vi "시리얼 테스트.vi"(11 "Serial Port":refnum<visa-resource-name>="COM6") -> ()   [LabVIEW 2015]
doc: "Use this template to create an application that executes repeatedly until you click the Stop button. This template polls the state of the Stop button and does not use events. Use the Top-Level Application template (not available in the Base package) to create a single-loop application with event handling."
uses:
  <vilib>/Utility/config.llb/Read Key (String).vi
  <vilib>/Utility/config.llb/Read Key (U32).vi
  <vilib>/Utility/config.llb/Read Key (Double).vi
  <vilib>/Utility/config.llb/Read Key (Boolean).vi
  <vilib>/Instr/_visa.llb/VISA Configure Serial Port (Instr).vi
  <vilib>/Utility/config.llb/Write Key (String).vi
  <vilib>/Utility/config.llb/Write Key (I32).vi
  <vilib>/Utility/config.llb/Write Key (Double).vi
  <vilib>/Utility/config.llb/Write Key (Boolean).vi
  <vilib>/Utility/config.llb/NI_LVConfig.lvlib
panel:
  out "수신 플래그":bool
  out "수신 버퍼 배열":u8[](array[numeric])=[79, 75, 43, 68, 73, 83, 67, 83, 79, 75, 43, 68, 73, 83, 51, 58, 54, 70, 55, 56, 55, 52, 54, 56, 50, 54, 57, 67, 79, 75, 43, 78, 65, 77, 69, 58, 71, 13, 10, 79, 75, 43, 68, 73, 83, 67, 69, 79, 75, 43, 68, 73, 83, 67, 83, 79, 75, 43, 68, 73, 83, 49, 58, 69, 50, 67, 70, 55, 57, 67, 69, 54, 68, 48, 49, 79, 75, 43, 78, 65, 77, 69, 58, 79, 117, 114, 67, 104, 97, 114, 97, 99, 116, 101, 114, 105, 115, 116, 105, 13, 10, 79, 75, 43, 68, 73, 83, 67, 69, 79, 75, 43, 68, 73, 83, 67, 83, 79, 75, 43, 68, 73, 83, 49, 58, 69, 50, 67, 70, 55, 57, 67, 69, 54, 68, 48, 49, 79, 75, 43, 78, 65, 77, 69, 58, 79, 117, 114, 67, 104, 97, 114, 97, 99, 116, 101, 114, 105, 115, 116, 105, 13, 10, 79, 75, 43, 68, 73, 83, 67, 69, 79, 75, 43, 71, 101, 116, 58, 48, 120, 70, 70, 69, 48, 79, 75, 43, 83, 101, 116, 58, 48, 120, 70, 48, 48, 68, 79, 75, 43, 71, 101, 116, 58, 48, 120, 70, 48, 48, 68, 79, 75, 43, 68, 73, 83, 73, 83, 79, 75, 43, 68, 73, 83, 67, 58, 48, 48, 48, 48, 48, 48, 48, 48, 58, 48, 48, 48, 48, 48, 48, 48, 48, 48, 48, 48, 48, 48, 48, 48, 48, 48, 48, 48, 48, 48, 48, 48, 48, 48, 48, 48, 48, 48, 48, 48, 48, 58, 48, 48, 48, 48, 48, 48, 48, 48, 48, 48, 58, 69, 50, 67, 70, 55, 57, 67, 69, 54, 68, 48, 49, 58, 45, 48, 51, 54, 79, 75, 43, 68, 73, 83, 67, 58, 48, 48, 48, 48, 48, 48, 48, 48, 58, 48, 48, 48, 48, 48, 48, 48, 48, 48, 48, 48, 48, 48, 48, 48, 48, 48, 48, 48, 48, 48, 48, 48, 48, 48, 48, 48, 48, 48, 48, 48, 48, 58, 48, 48, 48, 48, 48, 48, 48, 48, 48, 48, 58, 69, 50, 67, 70, 55, 57, 67, 69, 54, 68, 48, 49, 58, 45, 48, 51, 54, 79, 75, 43, 68, 73, 83, 67, 69, 79, 75, 43, 68, 73, 83, 67, 83, 79, 75, 43, 68, 73, 83, 49, 58, 69, 50, 67, 70, 55, 57, 67, 69, 54, 68, 48, 49, 79, 75, 43, 78, 65, 77, 69, 58, 79, 117, 114, 67, 104, 97, 114, 97, 99, 116, 101, 114, 105, 115, 116, 105, 13, 10, 79, 75, 43, 68, 73, 83, 67, 69, 79, 75, 43, 67, 79, 78, 78, 48, 79, 75, 43, 67, 79, 78, 78, 79, 75, 43, 76, 79, 83, 84, 79, 75, 79, 75, 79, 75]
  in  "Serial Port 동작":refnum<visa-resource-name>="COM6"
  in  "수신 텍스트 속성":enum16{"Normal", "'\\' code", "Password", "Hex"}(ring) caption="Display Style"
  in  "Pause":bool
  in  "Transmit New line":enum16{"None", "LF", "CR", "CR+LF"}(ring)
  in  "Baudrate(BPS)":T1(ring)=enum."9600"
  out "연속전송 타이머":u64=18183062
  in  "Interval(s)":dbl(slide)=0.1 min=0.001 max=5.0 step=0.001 scale=0.1..5.0
  in  "Clear":bool
  in  "포트 연결":bool=TRUE
  in  "TxD 14":string="aaaaaaa"
  in  "연속전송 1":bool
  in  "TxD 13":string="AT+CO1E2CF79CE6D01"
  in  "전송 13":bool
  in  "TxD 12":string="AT+CONN2"
  in  "전송 12":bool
  in  "TxD 11":string="AT+CONN0"
  in  "전송 11":bool
  in  "TxD 10":string="AT+DISI?"
  in  "전송 10":bool
  in  "TxD 9":string="AT+DISC?"
  in  "전송 9":bool
  in  "TxD 8":string="AT+VERS?"
  in  "전송 8":bool
  in  "TxD 7":string="AT+UUID?"
  in  "전송 7":bool
  in  "TxD 6":string="AT+UUID0xF00D"
  in  "전송 6":bool
  in  "TxD 5":string="AT+IBEA1"
  in  "전송 5":bool
  in  "TxD 4":string="AT+SHOW1"
  in  "전송 4":bool
  in  "TxD 3":string="AT+ROLE1"
  in  "전송 3":bool
  in  "TxD 2":string="AT+IMME1"
  in  "전송 2":bool
  in  "전송 1":bool
  in  "TxD 1":string="AT"
  in  "Program Exit":bool=TRUE
  out "Receive data":string="OK+DISCSOK+DIS3:6F787468269COK+NAME:G\r\nOK+DISCEOK+DISCSOK+DIS1:E2CF79CE6D01OK+NAME:OurCharacteristi\r\nOK+DISCEOK+DISCSOK+DIS1:E2CF79CE6D01OK+NAME:OurCharacteristi\r\nOK+DISCEOK+Get:0xFFE0OK+Set:0xF00DOK+Get:0xF00DOK+DISISOK+DISC:00000000:00000000000000000000000000000000:0000000000:E2CF79CE6D01:-036OK+DISC:00000000:00000000000000000000000000000000:0000000000:E2CF79CE6D01:-036OK+DISCEOK+DISCSOK+DIS1:E2CF79CE6D01OK+NAME:OurCharacteristi\r\nOK+DISCEOK+CONN0OK+CONNOK+LOSTOKOKOK"
  # "Serial Terminal"
  # "141126"
  # "Transmit"
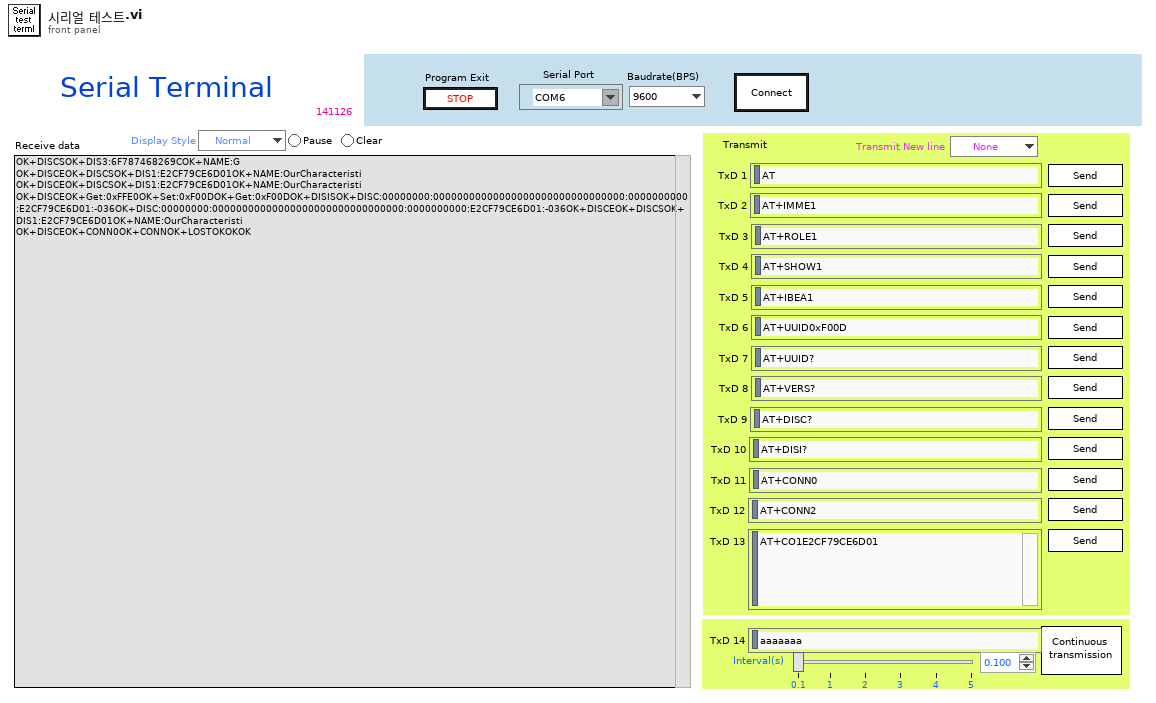
[diagram p1: front panel]
types:
  T1 = enum16{"110", "300", "600", "1200", "2400", "4800", "7200", "9600", "14400", "19200", "38400", "57600", "115200", "128000"}
  T2 = typedef "NI_LVConfig.lvlib/Config Data RefNum.ctl" = refnum<k1>
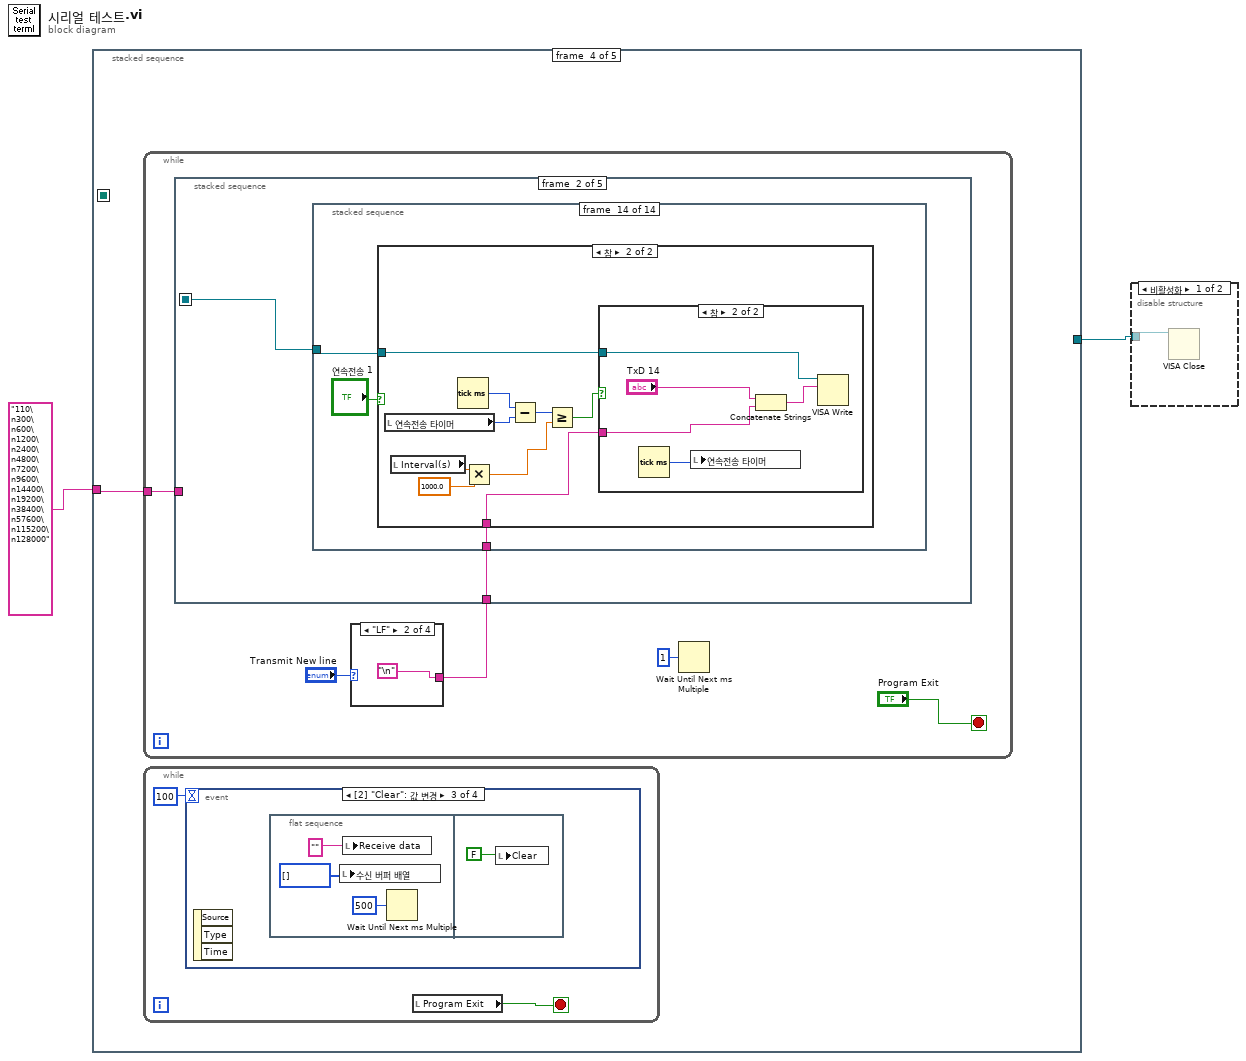
[diagram p0: block diagram]
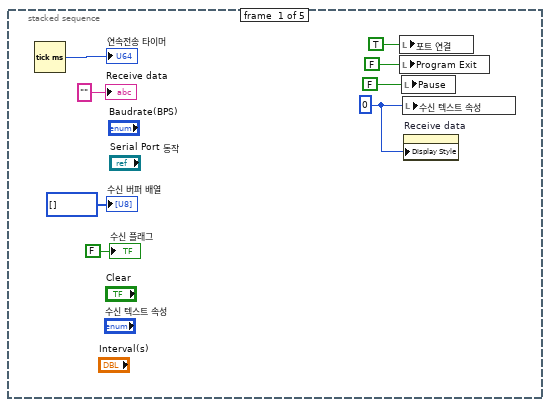
[diagram p3: hidden frame]
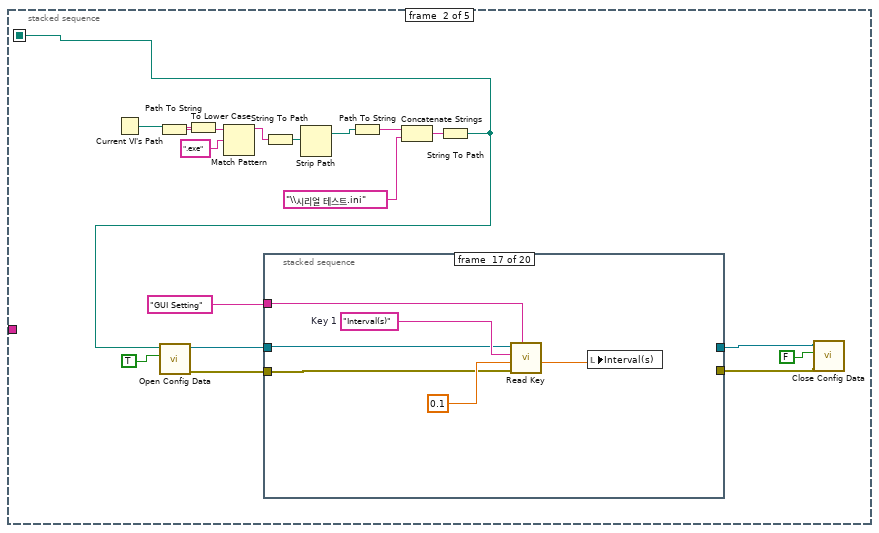
[diagram p4: hidden frame]
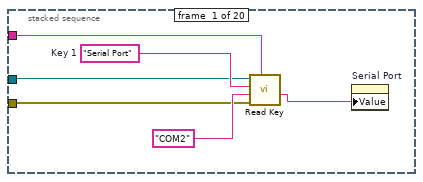
[diagram p5: hidden frame]
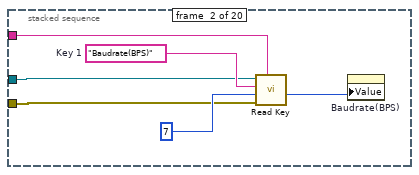
[diagram p6: hidden frame]
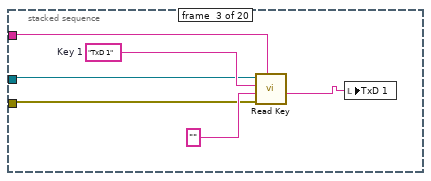
[diagram p7: hidden frame]
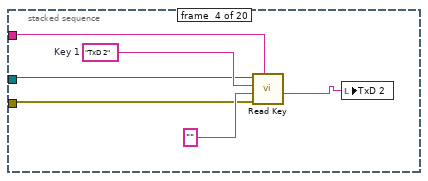
[diagram p8: hidden frame]
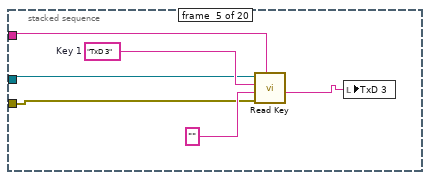
[diagram p9: hidden frame]
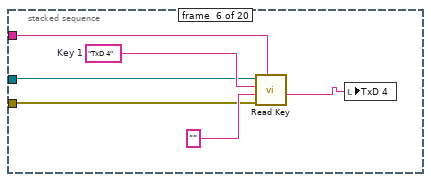
[diagram p10: hidden frame]
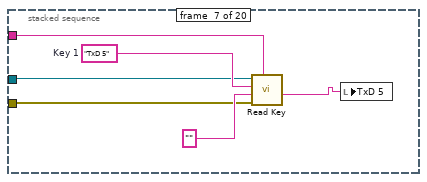
[diagram p11: hidden frame]
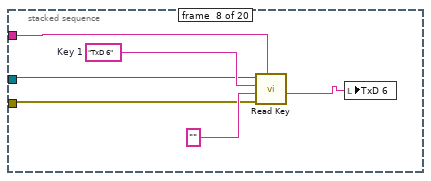
[diagram p12: hidden frame]
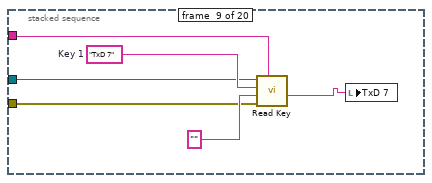
[diagram p13: hidden frame]
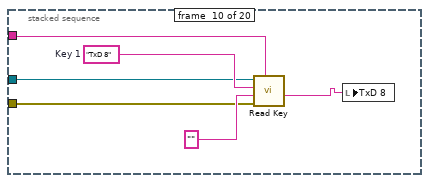
[diagram p14: hidden frame]
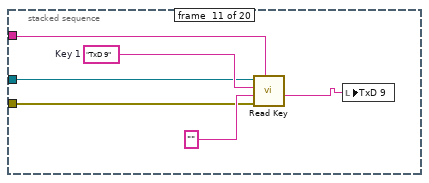
[diagram p15: hidden frame]
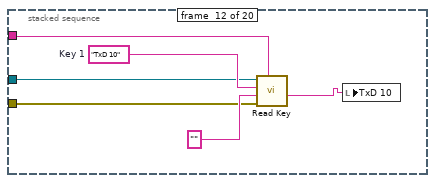
[diagram p16: hidden frame]
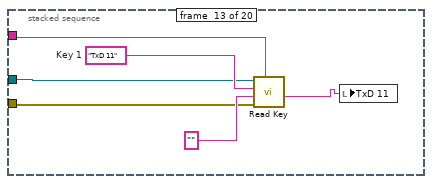
[diagram p17: hidden frame]
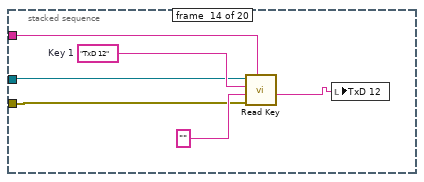
[diagram p18: hidden frame]
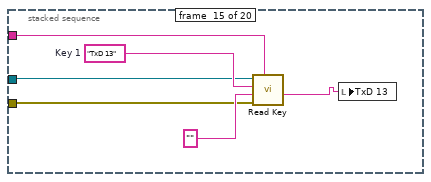
[diagram p19: hidden frame]
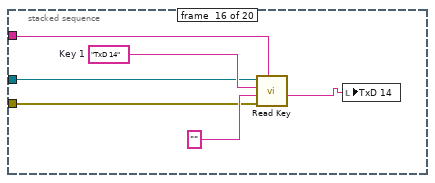
[diagram p20: hidden frame]
diagram:
  n1 = stacked-sequence {
    seq-local: [_ w11 _ _ _] -> [_ _ _ _ w350]
    tunnel: [_ _ _ _ w356] -> w2
    tunnel: "110\n300\n600\n1200\n2400\n4800\n7200\n9600\n14400\n19200\n38400\n57600\n115200\n128000" ("message") -> [_ _ w150 w158 _]
    frame #0 {
      w3 = 0
      n2 = Tick Count (ms)() -> (millisecond timer value=→"연속전송 타이머":u32)
      n3 = local write "포트 연결"(TRUE ("포트 연결")) -> ()
      n4 = local write "Program Exit"(FALSE ("프로그램 종료")) -> ()
      n5 = local write "Pause"(FALSE ("수신거부")) -> ()
      n6 = local write "수신 텍스트 속성"(w3) -> ()
      n7 = property on="Receive data" class="Str"("Display Style"=w3) -> ()  [unwired: 2 in, 2 out]
      "Receive data" <- "" ("수신 문자열")
      "수신 버퍼 배열" <- u8[] [] ("부호없는 바이트 배열")
      "수신 플래그" <- FALSE ("수신 플래그")
    }
    frame #1 {
      n8 = Current VI's Path() -> (path=w26:path)
      n9 = Path To String(path=w26) -> (string=w25:string)
      n10 = To Lower Case(string=w25) -> (all lower case string=w23:string)
      n11 = Match Pattern(string=w23, regular expression=".exe" ("search string")) -> (before substring=w22:string)  [unwired: 4 out]
      n12 = String To Path(string=w22) -> (path=w21:path)
      n13 = Strip Path(path=w21) -> (stripped path=w20:path)  [unwired: 1 out]
      n14 = Path To String(path=w20) -> (string=w19:string)
      n15 = Concatenate Strings(w19, "\\시리얼 테스트.ini" ("search string/char (-)")) -> (w28:string)
      n16 = String To Path(string=w28) -> (path=w11:path)
      n17 = call <vilib>:"Open Config Data.vi"("create file if necessary (T)"=TRUE, "configuration file path"=w11) -> ("error out"=w16:errorcluster, "refnum"=w15:T2)  [unwired: 7 in, 1 out]
      n18 = stacked-sequence {
        tunnel: "GUI Setting" ("section") -> [w32 w38 w43 w49 w55 w61 w67 w73 w79 w85 w91 w97 w103 w109 w115 w121 w127 w133 w139 _]
        tunnel: w15 -> [w31 w36 w42 w48 w54 w60 w66 w72 w78 w84 w90 w96 w102 w108 w114 w120 w126 w132 w138 w144]
        tunnel: w16 -> [w30 w35 w41 w47 w53 w59 w65 w71 w77 w83 w89 w95 w101 w107 w113 w119 w125 w131 w137 w143]
        tunnel: [_ _ _ _ _ _ _ _ _ _ _ _ _ _ _ _ _ _ _ w144] -> w17
        tunnel: [_ _ _ _ _ _ _ _ _ _ _ _ _ _ _ _ _ _ _ w143] -> w18
        frame #0 {
          w34 = "Serial Port"  # Key 1
          n19 = call-poly <vilib>:"Read Key.vi"("section"=w32, "error in (no error)"=w30, "default value"="COM2" ("output string"), "key"=w34, "refnum"=w31) -> ("value"=w29:string)  [unwired: 3 in, 3 out]
          n20 = property on="Serial Port" class="VISAName"("Value"=w29) -> ()  [unwired: 2 in, 2 out]
        }
        frame #1 {
          w39 = "Baudrate(BPS)"  # Key 1
          n21 = call-poly <vilib>:"Read Key.vi"("section"=w38, "error in (no error)"=w35, "default value"=u32 7, "key"=w39, "refnum"=w36) -> ("value"=w37:u32)  [unwired: 3 in, 3 out]
          n22 = property on="Baudrate(BPS)" class="Enum (엄격한)"("Value"=w37) -> ()  [unwired: 2 in, 2 out]
        }
        frame #2 {
          w45 = "TxD 1"  # Key 1
          n23 = call-poly <vilib>:"Read Key.vi"("section"=w43, "error in (no error)"=w41, "default value"="" ("output string"), "key"=w45, "refnum"=w42) -> ("value"=w46:string)  [unwired: 3 in, 3 out]
          n24 = local write "TxD 1"(w46) -> ()
        }
        frame #3 {
          w51 = "TxD 2"  # Key 1
          n25 = call-poly <vilib>:"Read Key.vi"("section"=w49, "error in (no error)"=w47, "default value"="" ("output string"), "key"=w51, "refnum"=w48) -> ("value"=w52:string)  [unwired: 3 in, 3 out]
          n26 = local write "TxD 2"(w52) -> ()
        }
        frame #4 {
          w57 = "TxD 3"  # Key 1
          n27 = call-poly <vilib>:"Read Key.vi"("section"=w55, "error in (no error)"=w53, "default value"="" ("output string"), "key"=w57, "refnum"=w54) -> ("value"=w58:string)  [unwired: 3 in, 3 out]
          n28 = local write "TxD 3"(w58) -> ()
        }
        frame #5 {
          w63 = "TxD 4"  # Key 1
          n29 = call-poly <vilib>:"Read Key.vi"("section"=w61, "error in (no error)"=w59, "default value"="" ("output string"), "key"=w63, "refnum"=w60) -> ("value"=w64:string)  [unwired: 3 in, 3 out]
          n30 = local write "TxD 4"(w64) -> ()
        }
        frame #6 {
          w69 = "TxD 5"  # Key 1
          n31 = call-poly <vilib>:"Read Key.vi"("section"=w67, "error in (no error)"=w65, "default value"="" ("output string"), "key"=w69, "refnum"=w66) -> ("value"=w70:string)  [unwired: 3 in, 3 out]
          n32 = local write "TxD 5"(w70) -> ()
        }
        frame #7 {
          w75 = "TxD 6"  # Key 1
          n33 = call-poly <vilib>:"Read Key.vi"("section"=w73, "error in (no error)"=w71, "default value"="" ("output string"), "key"=w75, "refnum"=w72) -> ("value"=w76:string)  [unwired: 3 in, 3 out]
          n34 = local write "TxD 6"(w76) -> ()
        }
        frame #8 {
          w81 = "TxD 7"  # Key 1
          n35 = call-poly <vilib>:"Read Key.vi"("section"=w79, "error in (no error)"=w77, "default value"="" ("output string"), "key"=w81, "refnum"=w78) -> ("value"=w82:string)  [unwired: 3 in, 3 out]
          n36 = local write "TxD 7"(w82) -> ()
        }
        frame #9 {
          w87 = "TxD 8"  # Key 1
          n37 = call-poly <vilib>:"Read Key.vi"("section"=w85, "error in (no error)"=w83, "default value"="" ("output string"), "key"=w87, "refnum"=w84) -> ("value"=w88:string)  [unwired: 3 in, 3 out]
          n38 = local write "TxD 8"(w88) -> ()
        }
        frame #10 {
          w93 = "TxD 9"  # Key 1
          n39 = call-poly <vilib>:"Read Key.vi"("section"=w91, "error in (no error)"=w89, "default value"="" ("output string"), "key"=w93, "refnum"=w90) -> ("value"=w94:string)  [unwired: 3 in, 3 out]
          n40 = local write "TxD 9"(w94) -> ()
        }
        frame #11 {
          w99 = "TxD 10"  # Key 1
          n41 = call-poly <vilib>:"Read Key.vi"("section"=w97, "error in (no error)"=w95, "default value"="" ("output string"), "key"=w99, "refnum"=w96) -> ("value"=w100:string)  [unwired: 3 in, 3 out]
          n42 = local write "TxD 10"(w100) -> ()
        }
        frame #12 {
          w105 = "TxD 11"  # Key 1
          n43 = call-poly <vilib>:"Read Key.vi"("section"=w103, "error in (no error)"=w101, "default value"="" ("output string"), "key"=w105, "refnum"=w102) -> ("value"=w106:string)  [unwired: 3 in, 3 out]
          n44 = local write "TxD 11"(w106) -> ()
        }
        frame #13 {
          w111 = "TxD 12"  # Key 1
          n45 = call-poly <vilib>:"Read Key.vi"("section"=w109, "error in (no error)"=w107, "default value"="" ("output string"), "key"=w111, "refnum"=w108) -> ("value"=w112:string)  [unwired: 3 in, 3 out]
          n46 = local write "TxD 12"(w112) -> ()
        }
        frame #14 {
          w117 = "TxD 13"  # Key 1
          n47 = call-poly <vilib>:"Read Key.vi"("section"=w115, "error in (no error)"=w113, "default value"="" ("output string"), "key"=w117, "refnum"=w114) -> ("value"=w118:string)  [unwired: 3 in, 3 out]
          n48 = local write "TxD 13"(w118) -> ()
        }
        frame #15 {
          w123 = "TxD 14"  # Key 1
          n49 = call-poly <vilib>:"Read Key.vi"("section"=w121, "error in (no error)"=w119, "default value"="" ("output string"), "key"=w123, "refnum"=w120) -> ("value"=w124:string)  [unwired: 3 in, 3 out]
          n50 = local write "TxD 14"(w124) -> ()
        }
        frame #16 {
          w128 = "Interval(s)"  # Key 1
          n51 = call-poly <vilib>:"Read Key.vi"("section"=w127, "error in (no error)"=w125, "default value"=0.1, "key"=w128, "refnum"=w126) -> ("value"=w129:dbl)  [unwired: 3 in, 3 out]
          n52 = local write "Interval(s)"(w129) -> ()
        }
        frame #17 {
          w134 = "Transmit New line"  # Key 1
          n53 = call-poly <vilib>:"Read Key.vi"("section"=w133, "error in (no error)"=w131, "default value"=u32 0, "key"=w134, "refnum"=w132) -> ("value"=w135:u32)  [unwired: 3 in, 3 out]
          n54 = local write "Transmit New line"(w135) -> ()
        }
        frame #18 {
          w140 = "Continuous transmission"  # Key 1
          n55 = call-poly <vilib>:"Read Key.vi"("section"=w139, "error in (no error)"=w137, "default value"=FALSE, "key"=w140, "refnum"=w138) -> ("value"=w141:bool)  [unwired: 3 in, 3 out]
          n56 = local write "연속전송 1"(w141) -> ()
        }
        frame #19 {
        }
      }
      n57 = call <vilib>:"Close Config Data.vi"("error in (no error)"=w18, "write file if changed (T)"=FALSE ("write configuration file? (T)"), "refnum"=w17) -> ()  [unwired: 9 out]
    }
    frame #2 {
      w146 = u16 10 items=["1.0"=10, "1.5"=15, "2.0"=20] ("stop bits (10: 1 bit)")
      n58 = property on="Baudrate(BPS)" class="Enum (엄격한)"() -> ("Value"=w147:T1)  [unwired: 2 in, 2 out]
      n59 = Pick Line(multi-line string=w150, line index=w147) -> (output string=w149:string)  [unwired: 1 out]
      n60 = Decimal String To Number(string=w149) -> (number=w148:i32)  [unwired: 3 out]
      n61 = call-poly "VISA Configure Serial Port"("VISA resource name"="Serial Port", "timeout (10sec)"=u32 10000, "Enable Termination\nChar (T)"=FALSE ("Enable Termination\nChar (T)"), "baud rate (9600)"=w148, "stop bits (10: 1 bit)"=w146) -> ("VISA resource name out"=w145:refnum<visa-resource-name>, "error out"=w154:errorcluster)  [unwired: 4 in, 5 out]
      n62 = Unbundle By Name(w154) -> ("status"=w151:bool)
      n63 = case shown="참" w151 {
        frame False {
        }
        frame True {
          n64 = local write "포트 연결"(FALSE ("포트 연결")) -> ()
          n65 = One Button Dialog(message="시리얼 포트가 잘못되었습니다.\n다시 확인해주세요...") -> ()  [unwired: 2 out]
          n66 = call <vilib>:"Beep.vi"() -> ()  [unwired: 3 in, 9 out]
        }
      }
      n67 = local write "Serial Port 동작"(w145) -> ()
    }
    frame #3 {
      n68 = while {
        tunnel: w158 -> [w170]
        stop <- "Program Exit" stop-if-true
        n69 = case shown="\"LF\"" "Transmit New line" {
          tunnel: ["" "\n" "\r" "\r\n"] -> w168
          frame "None", Default {
          }
          frame "LF" {
          }
          frame "CR" {
          }
          frame "CR+LF" {
          }
        }
        n70 = stacked-sequence {
          seq-local: [w176 _ _ _ _] -> [_ w177 w288 w313 _]
          tunnel: w170 -> [_ _ _ w314 _]
          tunnel: w168 -> [_ w178 _ _ _]
          frame #0 {
            n71 = local read "Serial Port 동작"() -> (w176:refnum<visa-resource-name>)
          }
          frame #1 {
            n72 = stacked-sequence {
              tunnel: w177 -> [w180 w187 w194 w201 w208 w215 w222 w229 w236 w243 w250 w257 w264 w271]
              tunnel: w178 -> [w179 w186 w193 w200 w207 w214 w221 w228 w235 w242 w249 w256 w263 w270]
              frame #0 {
                n73 = case shown="참" "전송 1" {
                  tunnel: w180 -> [_ w185]
                  tunnel: w179 -> [_ w182]
                  frame False {
                  }
                  frame True {
                    n74 = Concatenate Strings("TxD 1", w182) -> (w183:string)
                    n75 = VISA Write(VISA resource name=w185, write buffer=w183) -> ()  [unwired: 1 in, 3 out]
                  }
                }
              }
              frame #1 {
                n76 = case shown="거짓" "전송 2" {
                  tunnel: w187 -> [_ w192]
                  tunnel: w186 -> [_ w189]
                  frame False {
                  }
                  frame True {
                    n77 = Concatenate Strings("TxD 2", w189) -> (w190:string)
                    n78 = VISA Write(VISA resource name=w192, write buffer=w190) -> ()  [unwired: 1 in, 3 out]
                  }
                }
              }
              frame #2 {
                n79 = case shown="거짓" "전송 3" {
                  tunnel: w194 -> [_ w199]
                  tunnel: w193 -> [_ w196]
                  frame False {
                  }
                  frame True {
                    n80 = Concatenate Strings("TxD 3", w196) -> (w197:string)
                    n81 = VISA Write(VISA resource name=w199, write buffer=w197) -> ()  [unwired: 1 in, 3 out]
                  }
                }
              }
              frame #3 {
                n82 = case shown="거짓" "전송 4" {
                  tunnel: w201 -> [_ w206]
                  tunnel: w200 -> [_ w203]
                  frame False {
                  }
                  frame True {
                    n83 = Concatenate Strings("TxD 4", w203) -> (w204:string)
                    n84 = VISA Write(VISA resource name=w206, write buffer=w204) -> ()  [unwired: 1 in, 3 out]
                  }
                }
              }
              frame #4 {
                n85 = case shown="참" "전송 5" {
                  tunnel: w208 -> [_ w213]
                  tunnel: w207 -> [_ w210]
                  frame False {
                  }
                  frame True {
                    n86 = Concatenate Strings("TxD 5", w210) -> (w211:string)
                    n87 = VISA Write(VISA resource name=w213, write buffer=w211) -> ()  [unwired: 1 in, 3 out]
                  }
                }
              }
              frame #5 {
                n88 = case shown="거짓" "전송 6" {
                  tunnel: w215 -> [_ w220]
                  tunnel: w214 -> [_ w217]
                  frame False {
                  }
                  frame True {
                    n89 = Concatenate Strings("TxD 6", w217) -> (w218:string)
                    n90 = VISA Write(VISA resource name=w220, write buffer=w218) -> ()  [unwired: 1 in, 3 out]
                  }
                }
              }
              frame #6 {
                n91 = case shown="거짓" "전송 7" {
                  tunnel: w222 -> [_ w227]
                  tunnel: w221 -> [_ w224]
                  frame False {
                  }
                  frame True {
                    n92 = Concatenate Strings("TxD 7", w224) -> (w225:string)
                    n93 = VISA Write(VISA resource name=w227, write buffer=w225) -> ()  [unwired: 1 in, 3 out]
                  }
                }
              }
              frame #7 {
                n94 = case shown="거짓" "전송 8" {
                  tunnel: w229 -> [_ w234]
                  tunnel: w228 -> [_ w231]
                  frame False {
                  }
                  frame True {
                    n95 = Concatenate Strings("TxD 8", w231) -> (w232:string)
                    n96 = VISA Write(VISA resource name=w234, write buffer=w232) -> ()  [unwired: 1 in, 3 out]
                  }
                }
              }
              frame #8 {
                n97 = case shown="참" "전송 9" {
                  tunnel: w236 -> [_ w241]
                  tunnel: w235 -> [_ w238]
                  frame False {
                  }
                  frame True {
                    n98 = Concatenate Strings("TxD 9", w238) -> (w239:string)
                    n99 = VISA Write(VISA resource name=w241, write buffer=w239) -> ()  [unwired: 1 in, 3 out]
                  }
                }
              }
              frame #9 {
                n100 = case shown="참" "전송 10" {
                  tunnel: w243 -> [_ w248]
                  tunnel: w242 -> [_ w245]
                  frame False {
                  }
                  frame True {
                    n101 = Concatenate Strings("TxD 10", w245) -> (w246:string)
                    n102 = VISA Write(VISA resource name=w248, write buffer=w246) -> ()  [unwired: 1 in, 3 out]
                  }
                }
              }
              frame #10 {
                n103 = case shown="참" "전송 11" {
                  tunnel: w250 -> [_ w255]
                  tunnel: w249 -> [_ w252]
                  frame False {
                  }
                  frame True {
                    n104 = Concatenate Strings("TxD 11", w252) -> (w253:string)
                    n105 = VISA Write(VISA resource name=w255, write buffer=w253) -> ()  [unwired: 1 in, 3 out]
                  }
                }
              }
              frame #11 {
                n106 = case shown="참" "전송 12" {
                  tunnel: w257 -> [_ w262]
                  tunnel: w256 -> [_ w259]
                  frame False {
                  }
                  frame True {
                    n107 = Concatenate Strings("TxD 12", w259) -> (w260:string)
                    n108 = VISA Write(VISA resource name=w262, write buffer=w260) -> ()  [unwired: 1 in, 3 out]
                  }
                }
              }
              frame #12 {
                n109 = case shown="참" "전송 13" {
                  tunnel: w264 -> [_ w266]
                  tunnel: w263 -> [_ w269]
                  frame False {
                  }
                  frame True {
                    n110 = Concatenate Strings("TxD 13", w269) -> (w267:string)
                    n111 = VISA Write(VISA resource name=w266, write buffer=w267) -> ()  [unwired: 1 in, 3 out]
                  }
                }
              }
              frame #13 {
                n112 = case shown="참" "연속전송 1" {
                  tunnel: w271 -> [_ w282]
                  tunnel: w270 -> [_ w274]
                  frame False {
                    n113 = Tick Count (ms)() -> (millisecond timer value=w273:u32)
                    n114 = local write "연속전송 타이머"(w273) -> ()
                  }
                  frame True {
                    n115 = local read "연속전송 타이머"() -> (w280:u64)
                    n116 = local read "Interval(s)"() -> (w279:dbl)
                    n117 = Tick Count (ms)() -> (millisecond timer value=w281:u32)
                    n118 = Multiply(x=w279, y=1000.0) -> (x*y=w276:dbl)
                    n119 = Subtract(x=w281, y=w280) -> (x-y=w277:u64)
                    n120 = Greater Or Equal?(x=w277, y=w276) -> (x >= y?=w275:bool)
                    n121 = case shown="참" w275 {
                      tunnel: w282 -> [_ w287]
                      tunnel: w274 -> [_ w284]
                      frame False {
                      }
                      frame True {
                        n122 = Tick Count (ms)() -> (millisecond timer value=w285:u32)
                        n123 = local write "연속전송 타이머"(w285) -> ()
                        n124 = Concatenate Strings("TxD 14", w284) -> (w286:string)
                        n125 = VISA Write(VISA resource name=w287, write buffer=w286) -> ()  [unwired: 1 in, 3 out]
                      }
                    }
                  }
                }
              }
            }
          }
          frame #2 {
            n126 = property class="Instr"(reference=w288) -> (error out=w289:errorcluster, "Serial Settings:Number of Bytes at Serial Port"=w290:u32)  [unwired: 1 in, 1 out]
            n127 = case shown="에러" w289 {
              frame No Error {
              }
              frame Error {
                n128 = local write "포트 연결"(FALSE ("포트 연결")) -> ()
              }
            }
            n129 = Greater Than 0?(x=w290) -> (x > 0?=w291:bool)
            n130 = case shown="참" w291 {
              tunnel: w288 -> [_ w303]
              tunnel: w290 -> [_ w302]
              frame False {
                n131 = local read "수신 플래그"() -> (w293:bool)
                n132 = case shown="참" w293 {
                  frame False {
                  }
                  frame True {
                    n133 = local read "수신 버퍼 배열"() -> (w297:u8[])
                    n134 = Byte Array To String(unsigned byte array=w297) -> (string=w296:string)
                    n135 = local write "수신 플래그"(FALSE ("수신 플래그")) -> ()
                    n136 = property on="Receive data" class="Str"("Text.Scroll Position"=u32 4294967295) -> ()  [unwired: 2 in, 2 out]
                    n137 = local write "Receive data"(w296) -> ()
                  }
                }
              }
              frame True {
                n138 = local write "수신 플래그"(TRUE ("수신 플래그")) -> ()
                n139 = VISA Read(VISA resource name=w303, byte count=w302) -> (read buffer=w301:string)  [unwired: 1 in, 3 out]
                n140 = case shown="거짓" "Pause" {
                  tunnel: w301 -> [w312 _]
                  frame False {
                    w304 = 20000 ("y")
                    n141 = String To Byte Array(string=w312) -> (unsigned byte array=w310:u8[])
                    n142 = local read "수신 버퍼 배열"() -> (w311:u8[])
                    n143 = Insert Into Array(array=w311, new element=w310) -> (w307:u8[])  [unwired: 1 in]
                    n144 = Array Size(array=w307) -> (size(s)=w306:i32)
                    n145 = Subtract(x=w306, y=w304) -> (x-y=w305:i32)
                    n146 = Array Subset(array=w307, index=w305, length=w304) -> (w309:u8[])
                    n147 = Byte Array To String(unsigned byte array=w309) -> (string=w308:string)
                    n148 = local write "수신 버퍼 배열"(w307) -> ()
                    n149 = local write "Receive data"(w308) -> ()
                  }
                  frame True {
                  }
                }
                n150 = property on="Receive data" class="Str"("Text.Scroll Position"=u32 4294967295) -> ()  [unwired: 2 in, 2 out]
              }
            }
          }
          frame #3 {
            n151 = case shown="거짓" "포트 연결" {
              tunnel: w314 -> [w317 _]
              tunnel: w313 -> [w316 _]
              frame False {
                n152 = stacked-sequence {
                  seq-local: [_ w319 _] -> [_ _ w324]
                  tunnel: w316 -> [w318 _ _]
                  tunnel: w317 -> [_ _ w325]
                  frame #0 {
                    n153 = VISA Close(VISA resource name=w318) -> ()  [unwired: 1 in, 1 out]
                  }
                  frame #1 {
                    n154 = while {
                      tunnel: [w320] -> w319
                      stop <- w321 stop-if-true
                      n155 = local read "Program Exit"() -> (w320:bool)
                      n156 = local read "포트 연결"() -> (w322:bool)
                      n157 = Or(x=w322, y=w320) -> (x .or. y?=w321:bool)
                      n158 = Wait Until Next ms Multiple(millisecond multiple=u32 100) -> ()  [unwired: 1 out]
                    }
                  }
                  frame #2 {
                    n159 = case shown="거짓" w324 {
                      tunnel: w325 -> [w329 _]
                      frame False {
                        w328 = u16 10 items=["1.0"=10, "1.5"=15, "2.0"=20] ("stop bits (10: 1 bit)")
                        n160 = local read "Serial Port"() -> (w335:refnum<visa-resource-name>)
                        n161 = property on="Baudrate(BPS)" class="Enum (엄격한)"() -> ("Value"=w331:T1)  [unwired: 2 in, 2 out]
                        n162 = Pick Line(multi-line string=w329, line index=w331) -> (output string=w332:string)  [unwired: 1 out]
                        n163 = Decimal String To Number(string=w332) -> (number=w330:i32)  [unwired: 3 out]
                        n164 = call-poly "VISA Configure Serial Port"("VISA resource name"=w335, "timeout (10sec)"=u32 10000, "Enable Termination\nChar (T)"=FALSE ("Enable Termination\nChar (T)"), "baud rate (9600)"=w330, "data bits (8)"=u16 8, "stop bits (10: 1 bit)"=w328) -> ("VISA resource name out"=w327:refnum<visa-resource-name>, "error out"=w336:errorcluster)  [unwired: 3 in, 5 out]
                        n165 = Unbundle By Name(w336) -> ("status"=w333:bool)
                        n166 = case shown="참" w333 {
                          frame False {
                          }
                          frame True {
                            n167 = local write "포트 연결"(FALSE ("포트 연결")) -> ()
                            n168 = One Button Dialog(message="시리얼 포트가 잘못되었습니다.\n다시 확인해주세요...") -> ()  [unwired: 2 out]
                            n169 = call <vilib>:"Beep.vi"() -> ()  [unwired: 3 in, 9 out]
                          }
                        }
                        n170 = local write "Serial Port 동작"(w327) -> ()
                      }
                      frame True {
                      }
                    }
                  }
                }
              }
              frame True {
              }
            }
          }
          frame #4 {
            n171 = disable-structure shown="활성화" {
              frame Disabled {
                w341 = 1000000 ("y")
                n172 = local read "Receive data"() -> (w342:string)
                n173 = String Length(string=w342) -> (length=w340:i32)
                n174 = Greater?(x=w340, y=w341) -> (0:w343:bool)
                n175 = case shown="참" w343 {
                  tunnel: w342 -> [_ w348]
                  tunnel: w341 -> [_ w344]
                  tunnel: w340 -> [_ w345]
                  frame False {
                  }
                  frame True {
                    n176 = Subtract(x=w345, y=w344) -> (x-y=w346:i32)
                    n177 = String Subset(string=w348, offset (0)=w346) -> (substring=w347:string)  [unwired: 1 out]
                    n178 = local write "Receive data"(w347) -> ()
                  }
                }
              }
              frame Enabled {
              }
            }
          }
        }
        n179 = Wait Until Next ms Multiple(millisecond multiple=u32 1) -> ()  [unwired: 1 out]
      }
      n180 = while {
        stop <- w160 stop-if-true
        n181 = event shown="[2] \"Clear\": 값 변경" {
          selector: _ -> [_ _ _ _]
          dyn-events: _ -> [_ _ _ _]
          timeout: 100 -> [_ _ _ _]
          event Timeout {
            n182 = event-data() -> ()  [unwired: 1 in, 3 out]
          }
          event Panel Close? {
            w161 = TRUE ("버림?")
            n183 = event-data() -> ()  [unwired: 1 in, 3 out]
            n184 = local write "Program Exit"(w161) -> ()
            n185 = event-data("Discard?"=w161) -> ()  [unwired: 1 in, 1 out]
          }
          event "Clear": Value Change {
            n186 = event-data() -> ()  [unwired: 1 in, 3 out]
            n187 = flat-sequence {
              frame #0 {
                n188 = local write "수신 버퍼 배열"(u8[] [] ("부호없는 바이트 배열")) -> ()
                n189 = local write "Receive data"("" ("수신 문자열")) -> ()
                n190 = Wait Until Next ms Multiple(millisecond multiple=u32 500) -> ()  [unwired: 1 out]
              }
              frame #1 {
                n191 = local write "Clear"(FALSE ("화면 지우기")) -> ()
              }
            }
          }
          event "수신 텍스트 속성": Value Change {
            n192 = event-data() -> ("NewVal"=w166:enum16{"Normal", "'\\' code", "Password", "Hex"})  [unwired: 1 in, 2 out]
            n193 = property on="Receive data" class="Str"("Display Style"=w166) -> ()  [unwired: 2 in, 2 out]
          }
        }
        n194 = local read "Program Exit"() -> (w160:bool)
      }
    }
    frame #4 {
      n195 = call <vilib>:"Open Config Data.vi"("create file if necessary (T)"=TRUE, "configuration file path"=w350) -> ("error out"=w353:errorcluster, "refnum"=w352:T2)  [unwired: 1 in, 7 out]
      n196 = stacked-sequence {
        tunnel: "GUI Setting" ("section") -> [w360 w365 w369 w374 w379 w384 w389 w394 w399 w404 w409 w414 w419 w424 w429 w434 w439 w444 w449 _]
        tunnel: w352 -> [w359 w364 w368 w373 w378 w383 w388 w393 w398 w403 w408 w413 w418 w423 w428 w433 w438 w443 w448 w453]
        tunnel: w353 -> [w358 w363 w367 w372 w377 w382 w387 w392 w397 w402 w407 w412 w417 w422 w427 w432 w437 w442 w447 w452]
        tunnel: [_ _ _ _ _ _ _ _ _ _ _ _ _ _ _ _ _ _ _ w453] -> w354
        tunnel: [_ _ _ _ _ _ _ _ _ _ _ _ _ _ _ _ _ _ _ w452] -> w355
        frame #0 {
          w361 = "Serial Port"  # Key 1
          n197 = local read "Serial Port"() -> (w357:refnum<visa-resource-name>)
          n198 = call-poly <vilib>:"Write Key.vi"("section"=w360, "error in (no error)"=w358, "value"=w357, "key"=w361, "refnum"=w359) -> ()  [unwired: 1 in, 6 out]
        }
        frame #1 {
          w366 = "Baudrate(BPS)"  # Key 1
          n199 = property on="Baudrate(BPS)" class="Enum (엄격한)"() -> ("Value"=w362:T1)  [unwired: 2 in, 2 out]
          n200 = call-poly <vilib>:"Write Key.vi"("section"=w365, "error in (no error)"=w363, "value"=w362, "key"=w366, "refnum"=w364) -> ()  [unwired: 7 out]
        }
        frame #2 {
          w370 = "TxD 1"  # Key 1
          n201 = local read "TxD 1"() -> (w371:string)
          n202 = call-poly <vilib>:"Write Key.vi"("section"=w369, "error in (no error)"=w367, "value"=w371, "key"=w370, "refnum"=w368) -> ()  [unwired: 1 in, 6 out]
        }
        frame #3 {
          w375 = "TxD 2"  # Key 1
          n203 = local read "TxD 2"() -> (w376:string)
          n204 = call-poly <vilib>:"Write Key.vi"("section"=w374, "error in (no error)"=w372, "value"=w376, "key"=w375, "refnum"=w373) -> ()  [unwired: 1 in, 6 out]
        }
        frame #4 {
          w380 = "TxD 3"  # Key 1
          n205 = local read "TxD 3"() -> (w381:string)
          n206 = call-poly <vilib>:"Write Key.vi"("section"=w379, "error in (no error)"=w377, "value"=w381, "key"=w380, "refnum"=w378) -> ()  [unwired: 1 in, 6 out]
        }
        frame #5 {
          w385 = "TxD 4"  # Key 1
          n207 = local read "TxD 4"() -> (w386:string)
          n208 = call-poly <vilib>:"Write Key.vi"("section"=w384, "error in (no error)"=w382, "value"=w386, "key"=w385, "refnum"=w383) -> ()  [unwired: 1 in, 6 out]
        }
        frame #6 {
          w390 = "TxD 5"  # Key 1
          n209 = local read "TxD 5"() -> (w391:string)
          n210 = call-poly <vilib>:"Write Key.vi"("section"=w389, "error in (no error)"=w387, "value"=w391, "key"=w390, "refnum"=w388) -> ()  [unwired: 1 in, 6 out]
        }
        frame #7 {
          w395 = "TxD 6"  # Key 1
          n211 = local read "TxD 6"() -> (w396:string)
          n212 = call-poly <vilib>:"Write Key.vi"("section"=w394, "error in (no error)"=w392, "value"=w396, "key"=w395, "refnum"=w393) -> ()  [unwired: 1 in, 6 out]
        }
        frame #8 {
          w400 = "TxD 7"  # Key 1
          n213 = local read "TxD 7"() -> (w401:string)
          n214 = call-poly <vilib>:"Write Key.vi"("section"=w399, "error in (no error)"=w397, "value"=w401, "key"=w400, "refnum"=w398) -> ()  [unwired: 1 in, 6 out]
        }
        frame #9 {
          w405 = "TxD 8"  # Key 1
          n215 = local read "TxD 8"() -> (w406:string)
          n216 = call-poly <vilib>:"Write Key.vi"("section"=w404, "error in (no error)"=w402, "value"=w406, "key"=w405, "refnum"=w403) -> ()  [unwired: 1 in, 6 out]
        }
        frame #10 {
          w410 = "TxD 9"  # Key 1
          n217 = local read "TxD 9"() -> (w411:string)
          n218 = call-poly <vilib>:"Write Key.vi"("section"=w409, "error in (no error)"=w407, "value"=w411, "key"=w410, "refnum"=w408) -> ()  [unwired: 1 in, 6 out]
        }
        frame #11 {
          w415 = "TxD 10"  # Key 1
          n219 = local read "TxD 10"() -> (w416:string)
          n220 = call-poly <vilib>:"Write Key.vi"("section"=w414, "error in (no error)"=w412, "value"=w416, "key"=w415, "refnum"=w413) -> ()  [unwired: 1 in, 6 out]
        }
        frame #12 {
          w420 = "TxD 11"  # Key 1
          n221 = local read "TxD 11"() -> (w421:string)
          n222 = call-poly <vilib>:"Write Key.vi"("section"=w419, "error in (no error)"=w417, "value"=w421, "key"=w420, "refnum"=w418) -> ()  [unwired: 1 in, 6 out]
        }
        frame #13 {
          w425 = "TxD 12"  # Key 1
          n223 = local read "TxD 12"() -> (w426:string)
          n224 = call-poly <vilib>:"Write Key.vi"("section"=w424, "error in (no error)"=w422, "value"=w426, "key"=w425, "refnum"=w423) -> ()  [unwired: 1 in, 6 out]
        }
        frame #14 {
          w430 = "TxD 13"  # Key 1
          n225 = local read "TxD 13"() -> (w431:string)
          n226 = call-poly <vilib>:"Write Key.vi"("section"=w429, "error in (no error)"=w427, "value"=w431, "key"=w430, "refnum"=w428) -> ()  [unwired: 1 in, 6 out]
        }
        frame #15 {
          w435 = "TxD 14"  # Key 1
          n227 = local read "TxD 14"() -> (w436:string)
          n228 = call-poly <vilib>:"Write Key.vi"("section"=w434, "error in (no error)"=w432, "value"=w436, "key"=w435, "refnum"=w433) -> ()  [unwired: 1 in, 6 out]
        }
        frame #16 {
          w440 = "Interval(s)"  # Key 1
          n229 = local read "Interval(s)"() -> (w441:dbl)
          n230 = call-poly <vilib>:"Write Key.vi"("section"=w439, "error in (no error)"=w437, "value"=w441, "key"=w440, "refnum"=w438) -> ()  [unwired: 3 in, 4 out]
        }
        frame #17 {
          w445 = "Transmit New line"  # Key 1
          n231 = local read "Transmit New line"() -> (w446:enum16{"None", "LF", "CR", "CR+LF"})
          n232 = call-poly <vilib>:"Write Key.vi"("section"=w444, "error in (no error)"=w442, "value"=w446, "key"=w445, "refnum"=w443) -> ()  [unwired: 7 out]
        }
        frame #18 {
          w450 = "Continuous transmission"  # Key 1
          n233 = local read "연속전송 1"() -> (w451:bool)
          n234 = call-poly <vilib>:"Write Key.vi"("section"=w449, "error in (no error)"=w447, "value"=w451, "key"=w450, "refnum"=w448) -> ()  [unwired: 7 out]
        }
        frame #19 {
        }
      }
      n235 = call <vilib>:"Close Config Data.vi"("error in (no error)"=w355, "refnum"=w354) -> ()  [unwired: 1 in, 9 out]
      n236 = local read "Serial Port 동작"() -> (w356:refnum<visa-resource-name>)
    }
  }
  n237 = disable-structure shown="비활성화" {
    disable-tunnel: w2 -> [w454 _]
    frame Disabled {
      n238 = VISA Close(VISA resource name=w454) -> ()  [unwired: 1 in, 1 out]
    }
    frame Enabled {
    }
  }
